vi "Do.vi"(8 "error in":errorcluster, 10 "Actor in":refnum<class "Actor.lvclass">, 11 "O3 Valve MSG":refnum<class "O3 Valve MSG.lvclass">) -> (0 "error out":errorcluster, 2 "Actor out":refnum<class "Actor.lvclass">)   [LabVIEW 2014, in "Controller.lvlib" / "O3 Valve MSG.lvclass"]
doc: "(<B>Filename</B>: Actor Framework.lvlib:Message.lvclass:Do.vi)\n\nDefines what a message does when it is received by an actor. Generally, a message instructs an actor to invoke one of its methods. By default, this method does nothing. A child class must override it to define behavior. Create a child class by using the Actor Framework Message Maker dialog box."
uses:
  O3 Valve MSG.lvclass
  <vilib>/ActorFramework/Actor/Actor.lvclass
  Update Switch State MSG/Update Switch MSG.lvclass/Update Switch MSG.ctl
  Controller.lvclass
  SuperActor/Ex Nested.lvclass/Ex Nested.ctl
  SuperActor/Read Log Session.vi
  SuperActor/Read CVT Session.vi
  Update Switch State MSG/Read SwitchState.vi
  <vilib>/DAQmx/write.llb/DAQmx Write (Digital Bool 1Line 1Point).vi
  <userlib>/_Session Fwk/Session - Root.lvclass
  reusable/Session APIs/Session Log/System Log.lvclass
  reusable/Session APIs/CVT/CVT.lvclass
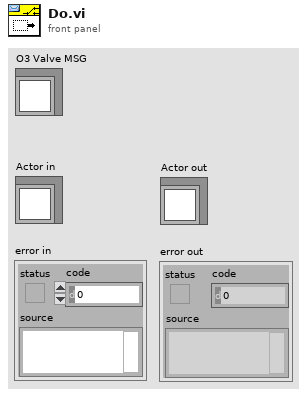
[diagram p1: front panel]
types:
  T1 = typedef "Session - Root.lvclass/Session Handle.ctl" = refnum<data-value>
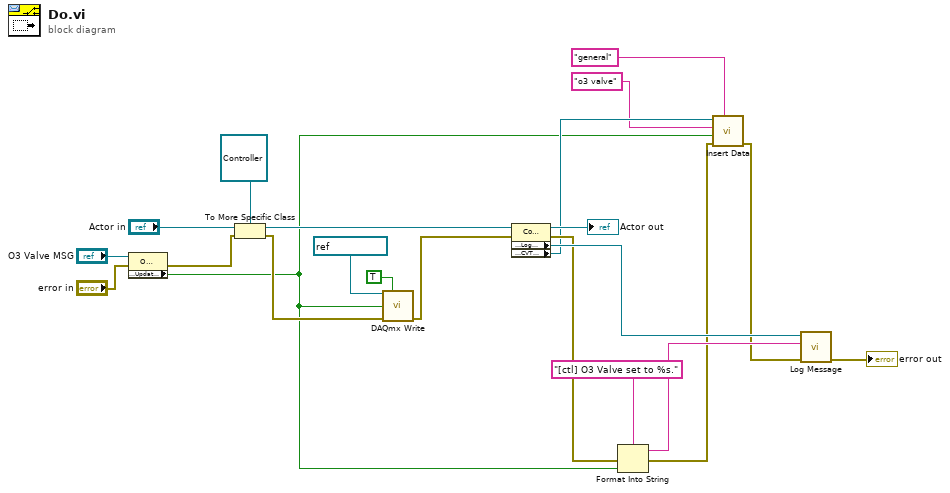
[diagram p0: block diagram]
diagram:
  n1 = property class="O3 Valve"(reference="O3 Valve MSG", error in="error in") -> (error out=w7:errorcluster, "Accessors:UpdateSw"=w3:bool)  [unwired: 1 out]
  n2 = To More Specific Class(target class=refnum<class "Controller.lvclass"> refnum ("Controller.lvlib:Controller"), reference="Actor in", error in=w7) -> (specific class reference=w17:refnum<class "Controller.lvclass">, error out=w18:errorcluster)
  n3 = call-poly <vilib>:"DAQmx Write.vi"("task/channels in"=refnum<k21> "O3 Valve", "auto start"=TRUE, "data"=w3, "error in"=w18) -> ("error out"=w16:errorcluster)  [unwired: 9 in, 2 out]
  n4 = property class="Controller"(reference=w17, error in=w16) -> (reference out=→"Actor out":refnum<class "Controller.lvclass">, error out=w13:errorcluster, "Accessors:Log Session"=w15:T1, "Accessors:CVT Session"=w6:T1)
  n5 = Format Into String(format string="[ctl] O3 Valve set to %s.", error in=w13, w3) -> (resulting string=w10:string, error out=w2:errorcluster)  [unwired: 1 in]
  n6 = call "Insert Data.vi"("Group"="general", "error in"=w2, "Data"=w3, "tag"="o3 valve", "CVT Session In"=w6) -> ("error out"=w1:errorcluster)  [unwired: 5 in, 1 out]
  n7 = call "Log Message.vi"("error in"=w1, "MSG In"=w10, "session in"=w15) -> ("error out"=→"error out":errorcluster)  [unwired: 7 in, 1 out]
